vi "Built Copyrights Text.vi"(0 "Description in":string, 5 "Licence Text":string, 11 "error in":errorcluster) -> (4 "Description out":string, 15 "error out":errorcluster)   [LabVIEW 2016, in "SLL Add Copyright.lvlib"]
uses:
  SLL Add Copyright.lvlib
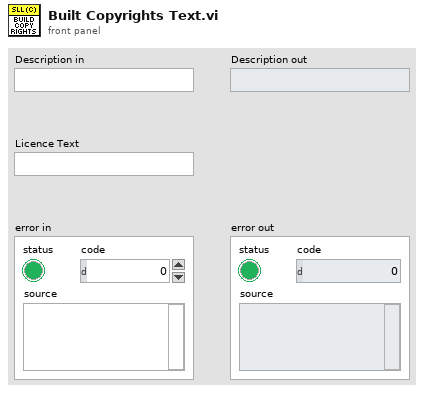
[diagram p1: front panel]
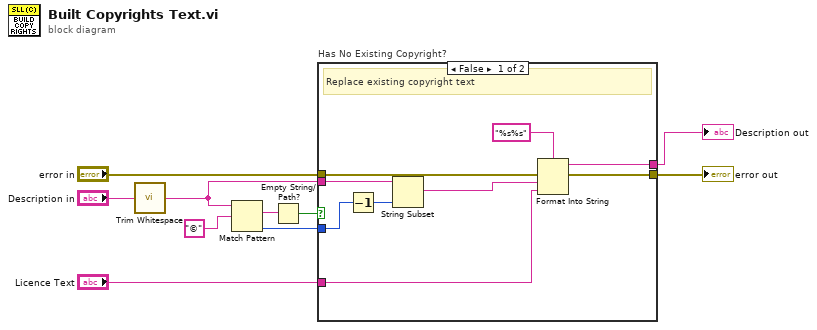
[diagram p0: block diagram]
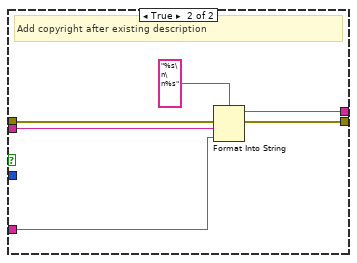
[diagram p2: hidden frame]
diagram:
  n1 = call <vilib>:"Trim Whitespace.vi"("string"="Description in") -> ("trimmed string"=w1:string)  [unwired: 1 in]
  n2 = Match Pattern(string=w1, regular expression="©") -> (match substring=w9:string, offset past match=w7:i32)  [unwired: 1 in, 2 out]
  n3 = Empty String/Path?(string/path=w9) -> (empty?=w8:bool)
  n4 = case "Has No Existing Copyright?" shown="False" w8 {
    tunnel: [w18 w24] -> w3
    tunnel: "error in" -> [w19 w25]
    tunnel: w1 -> [w15 w23]
    tunnel: [w16 w21] -> w2
    tunnel: w7 -> [w14 _]
    tunnel: "Licence Text" -> [w11 w20]
    frame False {
      # "Replace existing copyright text"
      n5 = Decrement(x=w14) -> (x-1=w12:i32)
      n6 = String Subset(string=w15, length (rest)=w12) -> (substring=w13:string)  [unwired: 1 in]
      n7 = Format Into String(format string="%s%s", error in=w19, w13, w11) -> (resulting string=w16:string, error out=w18:errorcluster)  [unwired: 1 in]
    }
    frame True {
      # "Add copyright after existing description"
      n8 = Format Into String(format string="%s\n\n%s", error in=w25, w23, w20) -> (resulting string=w21:string, error out=w24:errorcluster)  [unwired: 1 in]
    }
  }
  "error out" <- w3
  "Description out" <- w2
